vi "AD7609 Get Nsamples.vi"(0 "Number of Samples":u32, 1 "Sampling Rate (Hz)":dbl, 2 "Device Parameters":T1={"Timeout (ms)"=10000, "N channels bytes to read"=18, "Triggering mode"=0, "Input voltage range (V)"=1, "Oversampling ratio"=0} {"Oversampling ratio" items=["1", "2", "4", "8", "16", "32", "64"]; "Input voltage range (V)" items=["-5... +5 V", "-10... +10 V"]; "Triggering mode" items=["Software", "Hardware, falling edge, slave", "Hardware, rising edge, slave", "Hardware, falling edge, master", "Hardware, rising edge, master"]}, 4 "VISA resource name":refnum<visa-resource-name>) -> (5 "Channel volts":sgl[][](array[numeric]), 6 "Error out":errorcluster)   [LabVIEW 2022 SP3]
uses:
  AD7609/NA-Das_7609.ctl
  <vilib>/Instr/_visa.llb/VISA Open Access Mode.ctl
  Globals/Meas_global.vi
panel:
  out "Seconds in Vi":dbl
  out "Message":string
  out "Run Time(s)":dbl
  out "Channel data":sgl[][](graph)
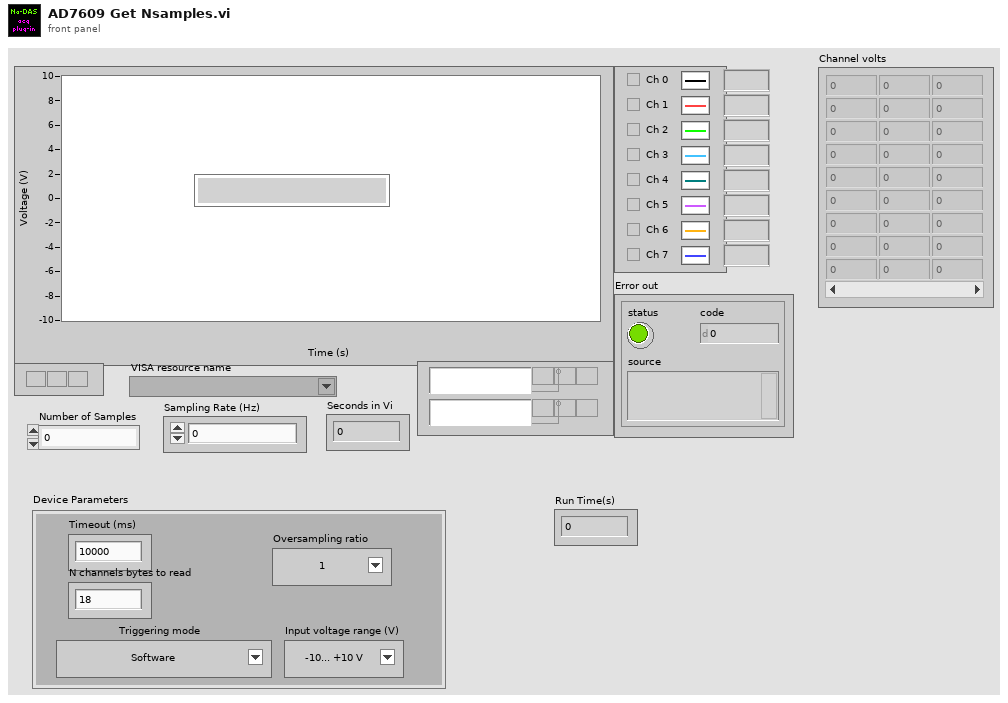
[diagram p1: front panel]
types:
  T1 = typedef "NA-Das_7609.ctl" = cluster{"Timeout (ms)":u32, "N channels bytes to read":u8, "Triggering mode":u8, "Input voltage range (V)":u8, "Oversampling ratio":u8}
  T2 = typedef "VISA Open Access Mode.ctl" = u32
  T3 = typedef "Setup.ctl" = enum16{"Run Program", "Show Setup", "Save Current Setup", "Setup Front Panel"}
  T4 = typedef "Rendezvous RefNum" = refnum<k1>
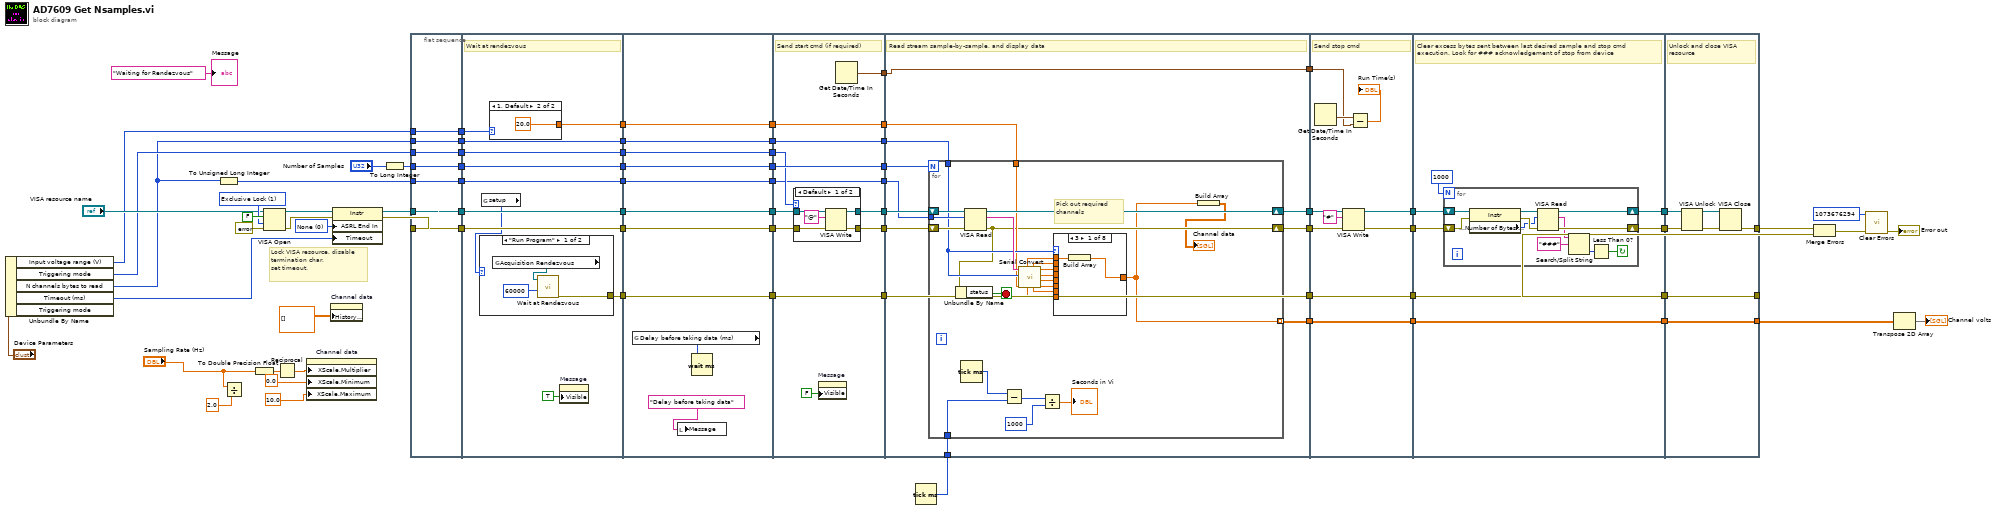
[diagram p0: block diagram]
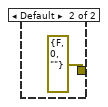
[diagram p2: hidden frame]
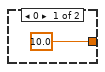
[diagram p3: hidden frame]
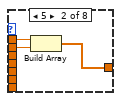
[diagram p5: hidden frame]
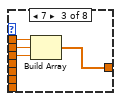
[diagram p6: hidden frame]
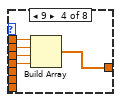
[diagram p7: hidden frame]
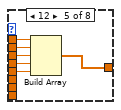
[diagram p8: hidden frame]
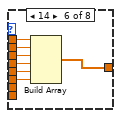
[diagram p9: hidden frame]
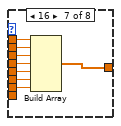
[diagram p10: hidden frame]
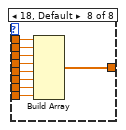
[diagram p11: hidden frame]
diagram:
  w58 = u16 0 items=["None", "Last Bit", "TermChar"] ("Serial Settings:End Mode for Reads")
  w75 = T2 1 items=["VISA Defaults"=0, "Exclusive Lock"=1, "Load Configured Settings"=4] ("Access Mode")
  # "Lock VISA resource, disable termination char,\nset timeout."
  n1 = Unbundle By Name("Device Parameters") -> ("Input voltage range (V)"=w21:u8, "Triggering mode"=w20:u8, "N channels bytes to read"=w19:u8, "Timeout (ms)"=w23:u32)  [unwired: 1 out]
  n2 = To Unsigned Long Integer(number=w19) -> (unsigned 32bit integer=w67:u32)
  n3 = Divide(x="Sampling Rate (Hz)", y=2.0) -> ()  [unwired: 1 out]
  n4 = To Double Precision Float(number="Sampling Rate (Hz)") -> (double precision float=w55:dbl)
  n5 = VISA Open(duplicate session (F)=FALSE, access mode=w75, error in (no error)=errorcluster {"status"=FALSE, "code"=0, "source"=""}, VISA resource name="VISA resource name") -> (VISA resource name=w62:refnum<visa-resource-name>, error out=w61:errorcluster)  [unwired: 1 in]
  n6 = Reciprocal(x=w55) -> (1/x=w56:dbl)
  n7 = property on="Channel data" class="WFChart (strict)"("XScale.Multiplier"=w56, "XScale.Minimum"=0.0 ("X Scale.Range:Minimum"), "XScale.Maximum"=10.0 ("X Scale.Range:Maximum")) -> ()  [unwired: 2 in, 2 out]
  n8 = property on="Channel data" class="WFChart (strict)"("History Data"=sgl[][] []) -> ()  [unwired: 2 in, 2 out]
  n9 = property class="Instr"(reference=w62, error in=w61, "ASRL End In"=w58, "Timeout"=w23) -> (reference out=w60:refnum<visa-resource-name>, error out=w59:errorcluster)
  n10 = To Long Integer(number="Number of Samples") -> (32bit integer=w69:i32)
  n11 = flat-sequence {
    tunnel: w19 -> [w79]
    tunnel: w21 -> [w80]
    tunnel: w67 -> [w81]
    tunnel: w20 -> [w78]
    tunnel: w69 -> [w82]
    tunnel: w60 -> [w83]
    tunnel: w59 -> [w84]
    tunnel: [w84] -> w33
    tunnel: [w83] -> w32
    tunnel: [w82] -> w31
    tunnel: [w78] -> w30
    tunnel: [w81] -> w29
    tunnel: [w80] -> w28
    tunnel: [w79] -> w27
    tunnel: [w95] -> w18
    tunnel: [w94] -> w16
    tunnel: [w93] -> w14
    tunnel: [w92] -> w12
    tunnel: [w91] -> w10
    tunnel: [w89] -> w8
    tunnel: [w88] -> w6
    tunnel: [w87] -> w4
    tunnel: w33 -> [w95]
    tunnel: w32 -> [w94]
    tunnel: w31 -> [w93]
    tunnel: w30 -> [w92]
    tunnel: w29 -> [w91]
    tunnel: w28 -> [w90]
    tunnel: w27 -> [w89]
    tunnel: w18 -> [w111]
    tunnel: [w111] -> w17
    tunnel: w16 -> [w110]
    tunnel: [w110] -> w15
    tunnel: w14 -> [w109]
    tunnel: [w109] -> w13
    tunnel: w12 -> [w108]
    tunnel: [w108] -> w11
    tunnel: w10 -> [w107]
    tunnel: [w107] -> w9
    tunnel: w8 -> [w106]
    tunnel: [w106] -> w7
    tunnel: w6 -> [w105]
    tunnel: [w105] -> w5
    tunnel: w4 -> [w104]
    tunnel: [w104] -> w3
    tunnel: [w121] -> w74
    tunnel: [w120] -> w71
    tunnel: [w119] -> w70
    tunnel: [w117] -> w68
    tunnel: [w116] -> w51
    tunnel: [w115] -> w45
    tunnel: w17 -> [w123]
    tunnel: w15 -> [w122]
    tunnel: w13 -> [w119]
    tunnel: w11 -> [w118]
    tunnel: w9 -> [w117]
    tunnel: w7 -> [w116]
    tunnel: w5 -> [w115]
    tunnel: w3 -> [w114]
    tunnel: [w114] -> w39
    tunnel: [w113] -> w34
    tunnel: w74 -> [w142]
    tunnel: [w141] -> w73
    tunnel: [w140] -> w72
    tunnel: w71 -> [w139]
    tunnel: w70 -> [w138]
    tunnel: w68 -> [w137]
    tunnel: w51 -> [w136]
    tunnel: [w135] -> w48
    tunnel: w45 -> [w134]
    tunnel: [w133] -> w40
    tunnel: w39 -> [w133]
    tunnel: [w132] -> w35
    tunnel: w34 -> [w132]
    tunnel: w1 -> [w131]
    tunnel: w73 -> [w219]
    tunnel: w72 -> [w220]
    tunnel: [w218] -> w65
    tunnel: [w217] -> w66
    tunnel: [w215] -> w49
    tunnel: w48 -> [w215]
    tunnel: [w214] -> w41
    tunnel: w40 -> [w214]
    tunnel: w35 -> [w212]
    tunnel: w66 -> [w224]
    tunnel: w65 -> [w227]
    tunnel: [w226] -> w64
    tunnel: [w225] -> w63
    tunnel: [w223] -> w50
    tunnel: w49 -> [w223]
    tunnel: [w222] -> w42
    tunnel: w41 -> [w222]
    tunnel: [w243] -> w53
    tunnel: w64 -> [w242]
    tunnel: w63 -> [w241]
    tunnel: w50 -> [w240]
    tunnel: [w240] -> w46
    tunnel: [w239] -> w43
    tunnel: w42 -> [w239]
    frame #0 {
    }
    frame #1 {
      # "Wait at rendezvous"
      n12 = global read "Meas_global.vi" "setup"() -> (w86:T3)
      n13 = case shown="\"Run Program\"" w86 {
        tunnel: [w98 errorcluster {"status"=FALSE, "code"=0, "source"=""} ("error out")] -> w87
        frame "Run Program" {
          n14 = global read "Meas_global.vi" "Acquisition Rendezvous"() -> (w97:T4)
          n15 = call <vilib>:"Wait at Rendezvous.vi"("ms timeout (-1)"=60000, "rendezvous"=w97) -> ("error out"=w98:errorcluster)  [unwired: 3 in, 2 out]
        }
        frame Default {
        }
      }
      n16 = case shown="1, Default" w90 {
        tunnel: [sgl 10.0 sgl 20.0] -> w88
        frame 0 {
        }
        frame 1, Default {
        }
      }
      n17 = property on="Message" class="Str"("Visible"=TRUE) -> ()  [unwired: 2 in, 2 out]
    }
    frame #2 {
      n18 = global read "Meas_global.vi" "Delay before taking data (ms)"() -> (w103:u32)
      n19 = local write "Message"("Delay before taking data" ("Message")) -> ()
      n20 = Wait (ms)(milliseconds to wait=w103) -> ()  [unwired: 1 out]
    }
    frame #3 {
      # "Send start cmd (if required)"
      n21 = case shown="Default" w118 {
        tunnel: w123 -> [w127 w129]
        tunnel: w122 -> [w126 w130]
        tunnel: [w125 w129] -> w121
        tunnel: [w124 w130] -> w120
        frame Default {
          n22 = VISA Write(VISA resource name=w126, write buffer="@", error in (no error)=w127) -> (VISA resource name out=w124:refnum<visa-resource-name>, error out=w125:errorcluster)  [unwired: 1 out]
        }
        frame 1, 2 {
        }
      }
      n23 = property on="Message" class="Str"("Visible"=FALSE) -> ()  [unwired: 2 in, 2 out]
      n24 = Get Date/Time In Seconds() -> (seconds since 1Jan1904=w113:timestamp)
    }
    frame #4 {
      # "Read stream sample-by-sample, and display data"
      n25 = for {
        N: w138 -> [_]
        shift-right: [w151] -> w141
        shift-left: w142 -> [w166]
        shift-right: [w165] -> w140
        shift-left: w139 -> [w164]
        tunnel: w137 -> [w155]
        tunnel: w136 -> [w154]
        tunnel: [w150] -> w135 mode=indexing
        tunnel: w134 -> [w153]
        tunnel: w131 -> [w146]
        stop <- w148 stop-if-true
        # "Pick out required channels"
        n26 = Tick Count (ms)() -> (millisecond timer value=w147:u32)
        n27 = VISA Read(VISA resource name=w164, byte count=w155, error in (no error)=w166) -> (VISA resource name out=w165:refnum<visa-resource-name>, read buffer=w156:string, error out=w151:errorcluster)  [unwired: 1 out]
        n28 = Unbundle By Name(w151) -> ("status"=w148:bool)
        n29 = Subtract(x=w147, y=w146) -> (x-y=w145:u32)
        n30 = call "Serial Convert.vi"("Range (V)"=w153, "N channels bytes to read"=w154, "Raw serial buffer"=w156) -> ("V6 (V)"=w159:sgl, "V5 (V)"=w160:sgl, "V4 (V)"=w161:sgl, "V3 (V)"=w162:sgl, "V7 (V)"=w158:sgl, "V2 (V)"=w152:sgl, "V8 (V)"=w157:sgl, "V1 (V)"=w163:sgl)  [unwired: 1 in]
        n31 = Divide(x=w145, y=u32 1000) -> (x/y=→"Seconds in Vi":dbl)
        n32 = case shown="3" w154 {
          tunnel: w163 -> [w168 w171 w175 w180 w186 w193 w201 w210]
          tunnel: w152 -> [_ w169 w174 w179 w185 w192 w200 w209]
          tunnel: w162 -> [_ _ w173 w178 w184 w191 w199 w208]
          tunnel: w161 -> [_ _ _ w177 w183 w190 w198 w207]
          tunnel: w160 -> [_ _ _ _ w182 w189 w197 w206]
          tunnel: w159 -> [_ _ _ _ _ w188 w196 w205]
          tunnel: w158 -> [_ _ _ _ _ _ w195 w204]
          tunnel: w157 -> [_ _ _ _ _ _ _ w203]
          tunnel: [w167 w170 w172 w176 w181 w187 w194 w202] -> w150
          frame 3 {
            n33 = Build Array(w168) -> (w167:sgl[])
          }
          frame 5 {
            n34 = Build Array(w171, w169) -> (w170:sgl[])
          }
          frame 7 {
            n35 = Build Array(w175, w174, w173) -> (w172:sgl[])
          }
          frame 9 {
            n36 = Build Array(w180, w179, w178, w177) -> (w176:sgl[])
          }
          frame 12 {
            n37 = Build Array(w186, w185, w184, w183, w182) -> (w181:sgl[])
          }
          frame 14 {
            n38 = Build Array(w193, w192, w191, w190, w189, w188) -> (w187:sgl[])
          }
          frame 16 {
            n39 = Build Array(w201, w200, w199, w198, w197, w196, w195) -> (w194:sgl[])
          }
          frame 18, Default {
            n40 = Build Array(w210, w209, w208, w207, w206, w205, w204, w203) -> (w202:sgl[])
          }
        }
        n41 = Build Array(w150) -> (→"Channel data":sgl[][])
      }
    }
    frame #5 {
      # "Send stop cmd"
      n42 = Get Date/Time In Seconds() -> (seconds since 1Jan1904=w213:timestamp)
      n43 = VISA Write(VISA resource name=w220, write buffer="#", error in (no error)=w219) -> (VISA resource name out=w218:refnum<visa-resource-name>, error out=w217:errorcluster)  [unwired: 1 out]
      n44 = Subtract(x=w213, y=w212) -> (x-y=→"Run Time(s)":dbl)
    }
    frame #6 {
      # "Clear excess bytes sent between last desired sample and stop cmd execution. Look for ### acknowledgement of stop from device"
      n45 = for {
        N: 1000 -> [_]
        shift-right: [w234] -> w226
        shift-left: w224 -> [w237]
        shift-right: [w233] -> w225
        shift-left: w227 -> [w238]
        stop <- w228 continue-if-true
        n46 = property class="Instr"(reference=w238, error in=w237) -> (reference out=w236:refnum<visa-resource-name>, error out=w235:errorcluster, "Serial Settings:Number of Bytes at Serial Port"=w229:u32)
        n47 = VISA Read(VISA resource name=w236, byte count=w229, error in (no error)=w235) -> (VISA resource name out=w233:refnum<visa-resource-name>, read buffer=w232:string, error out=w234:errorcluster)  [unwired: 1 out]
        n48 = Search/Split String(string=w232, search string/char (-)="###") -> (offset of match=w230:i32)  [unwired: 1 in, 2 out]
        n49 = Less Than 0?(x=w230) -> (x < 0?=w228:bool)
      }
    }
    frame #7 {
      # "Unlock and close VISA resource"
      n50 = VISA Unlock(8:w242, 11:w241) -> (0:w245:errorcluster, 3:w244:refnum<visa-resource-name>)
      n51 = VISA Close(VISA resource name=w244, error in (no error)=w245) -> (error out=w243:errorcluster)
    }
  }
  n52 = Tick Count (ms)() -> (millisecond timer value=w1:u32)
  n53 = Merge Errors(w53, w43) -> (w44:errorcluster)
  n54 = call <vilib>:"Clear Errors.vi"("error in (no error)"=w44, "specific error code to clear (0: all)"=1073676294) -> ("error out"=→"Error out":errorcluster)  [unwired: 4 in, 1 out]
  n55 = Transpose 2D Array(2D array=w46) -> (transposed array=→"Channel volts":sgl[][])
  "Message" <- "Waiting for Rendezvous" ("Message")
